vi "Test-SharedVariable1.vi"   [LabVIEW 2014]
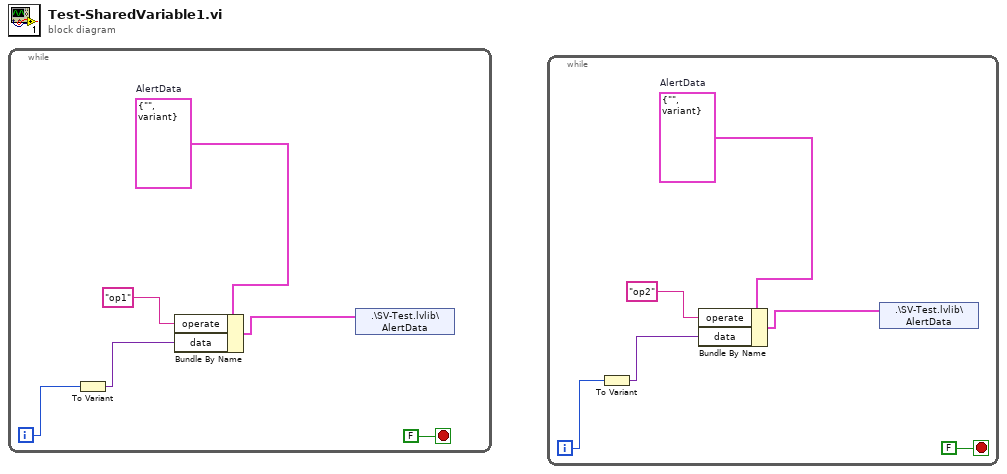
[diagram p0: block diagram]
diagram:
  n1 = while {
    i -> [w2]
    stop <- FALSE stop-if-true
    w5 = cluster{"operate":string, "data":variant} {"operate"="", "data"=variant}  # AlertData
    n2 = To Variant(anything=w2) -> (Variant=w1:variant)
    n3 = Bundle By Name(cluster=w5, "operate"="op1", "data"=w1) -> (w4:cluster{"operate":string, "data":variant})
    n4 = shared-variable ".\\SV-Test.lvlib\\AlertData"(w4) -> ()  [unwired: 1 in, 1 out]
  }
  n5 = while {
    i -> [w8]
    stop <- FALSE stop-if-true
    w9 = cluster{"operate":string, "data":variant} {"operate"="", "data"=variant}  # AlertData
    n6 = To Variant(anything=w8) -> (Variant=w12:variant)
    n7 = Bundle By Name(cluster=w9, "operate"="op2", "data"=w12) -> (w10:cluster{"operate":string, "data":variant})
    n8 = shared-variable ".\\SV-Test.lvlib\\AlertData"(w10) -> ()  [unwired: 1 in, 1 out]
  }
